vi "Send UDP Packet.vi"(8 "error in (no error)":errorcluster, 11 "Assert Message in":T1) -> (0 "error out":errorcluster)   [LabVIEW 2016, in "Assert API Components.lvlib" / "Log Assert Core.lvlib"]
doc: "Sends the message back over the UDP port to the main display with the relevant data"
uses:
  Log Assert Core.lvlib
  Message Data.ctl
  VI References.ctl
  <vilib>/Utility/config.llb/Read Key (String).vi
  <vilib>/Utility/config.llb/NI_LVConfig.lvlib
  Assert API Components.lvlib
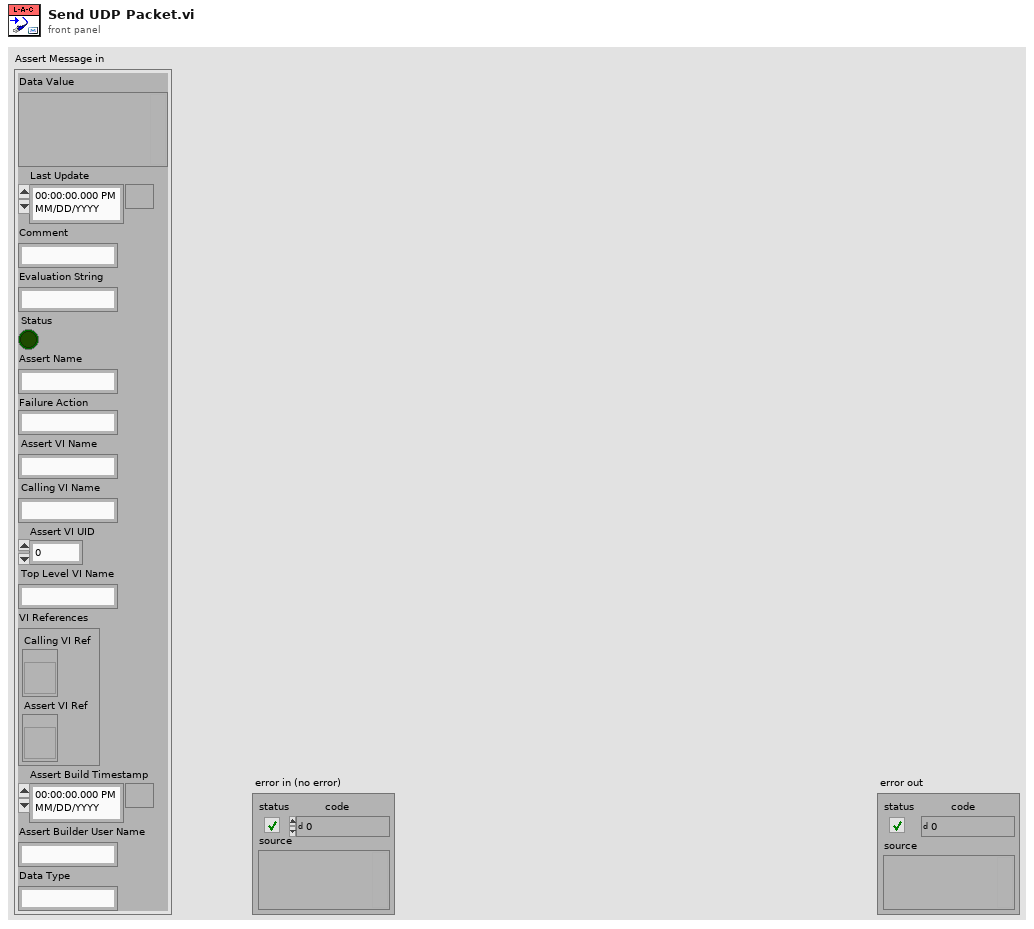
[diagram p1: front panel]
types:
  T1 = typedef "Assert API Components.lvlib/Message Data.ctl" = cluster{"Data Value":variant, "Last Update":timestamp, "Comment":string, "Evaluation String":string, "Status":bool, "Assert Name":string, "Failure Action":string, "Assert VI Name":string, "Calling VI Name":string, "Assert VI UID":i32, "Top Level VI Name":string, "VI References":T2, "Assert Build Timestamp":timestamp, "Assert Builder User Name":string, "Data Type":string}
  T2 = typedef "Assert API Components.lvlib/VI References.ctl" = cluster{"Calling VI Ref":refnum<vi>, "Assert VI Ref":refnum<vi>}
  T3 = typedef "NI_LVConfig.lvlib/Config Data RefNum.ctl" = refnum<k1>
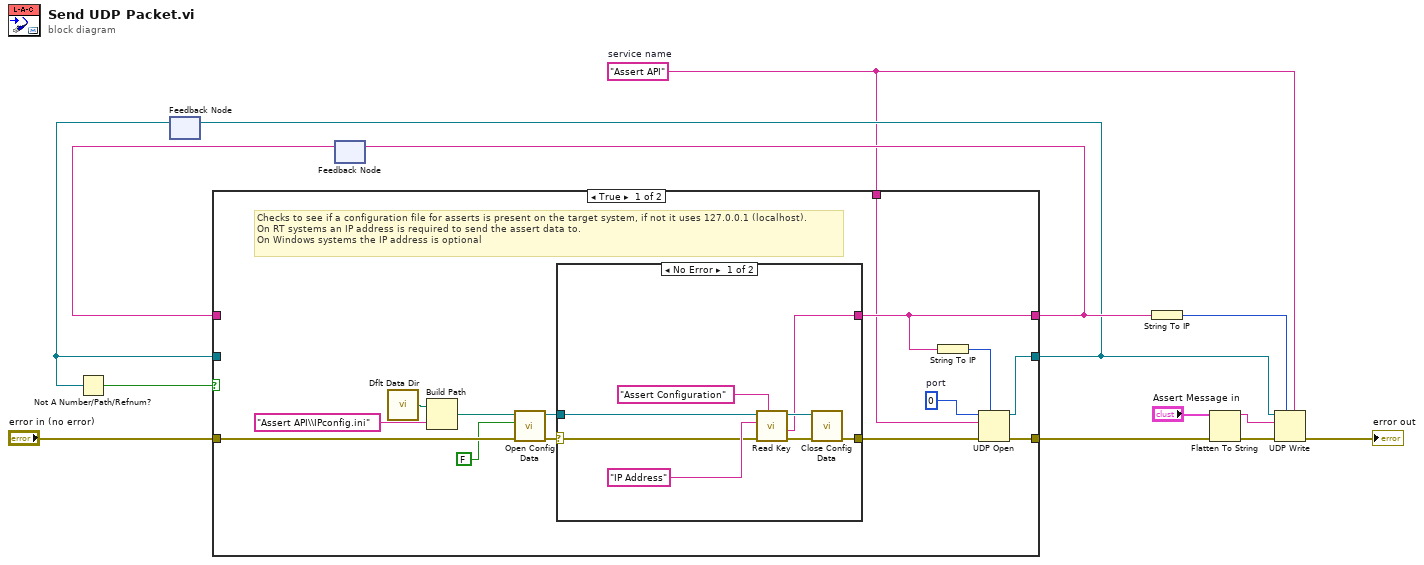
[diagram p0: block diagram]
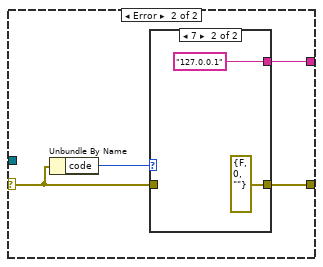
[diagram p2: hidden frame]
diagram:
  w1 = "Assert API"  # service name
  n1 = feedback #1() -> (w9:refnum<k16>)  [unwired: 1 in]
  n2 = Not A Number/Path/Refnum?(number/path/refnum=w9) -> (NaN/Path/Refnum?=w8:bool)
  n3 = feedback #2() -> (w7:string)  [unwired: 1 in]
  n4 = case shown="True" w8 {
    tunnel: [w25 w44] -> w3
    tunnel: "error in (no error)" -> [w24 w45]
    tunnel: [w26 w45] -> w2
    tunnel: w9 -> [_ w44]
    tunnel: [w15 w43] -> w5
    tunnel: w7 -> [_ w43]
    tunnel: w1 -> [w14 _]
    frame True {
      w27 = u16 0  # port
      # "Checks to see if a configuration file for asserts is present on the target system, if not it uses 127.0.0.1 (localhost).\nOn RT systems an IP address is required to send the assert data to.\nOn Windows systems the IP address is optional"
      n5 = call <vilib>:"Dflt Data Dir.vi"() -> ("App:Default Data Directory"=w23:path)
      n6 = Build Path(base path=w23, name or relative path="Assert API\\IPconfig.ini") -> (appended path=w21:path)
      n7 = call <vilib>:"Open Config Data.vi"("error in (no error)"=w24, "create file if necessary (T)"=FALSE, "configuration file path"=w21) -> ("error out"=w19:errorcluster, "refnum"=w18:T3)  [unwired: 6 in, 1 out]
      n8 = case shown="No Error" w19 {
        selector: w19 -> [w32 w37]
        tunnel: w18 -> [w33 _]
        tunnel: [w28 w38] -> w15
        tunnel: [w29 w36] -> w17
        frame No Error {
          n9 = call-poly <vilib>:"Read Key.vi"("section"="Assert Configuration", "error in (no error)"=w32, "key"="IP Address", "refnum"=w33) -> ("error out"=w30:errorcluster, "value"=w28:string, "refnum out"=w31:T3)  [unwired: 4 in, 1 out]
          n10 = call <vilib>:"Close Config Data.vi"("error in (no error)"=w30, "refnum"=w31) -> ("error out"=w29:errorcluster)  [unwired: 8 in, 1 out]
        }
        frame Error {
          n11 = Unbundle By Name(w37) -> ("code"=w39:i32)
          n12 = case shown="7" w39 {
            tunnel: [_ "127.0.0.1"] -> w38
            tunnel: w37 -> [w40 _]
            tunnel: [w40 errorcluster {"status"=FALSE, "code"=0, "source"=""} ("error IO")] -> w36
            frame Default {
            }
            frame 7 {
            }
          }
        }
      }
      n13 = String To IP(1:w15) -> (0:w16:u32)
      n14 = UDP Open(7:w16, 8:w17, 10:w14, 11:w27) -> (port=w25:refnum<k16>, 0:w26:errorcluster)  [unwired: 1 in, 1 out]
    }
    frame False {
    }
  }
  n15 = feedback-in #1(w3) -> ()
  n16 = feedback-in #2(w5) -> ()
  n17 = String To IP(1:w5) -> (0:w4:u32)
  n18 = Flatten To String(anything="Assert Message in", error in (no error)=w2) -> (data string=w12:string, error out=w11:errorcluster)  [unwired: 2 in, 1 out]
  n19 = UDP Write(address=w4, port or service name=w1, connection ID=w3, data in=w12, 8:w11) -> (error out=→"error out":errorcluster)  [unwired: 1 in, 1 out]
